vi "PH_Timing.calc GateGen Settings.vi"(5 "T2 [s]":i16 min=0 max=3000 step=100) -> (20 "Width Gate":dbl, 22 "Width T2":dbl, 24 "Delay Gate":dbl, 26 "Delay T2":dbl)   [LabVIEW 2014, in "PH_Timing.lvlib"]
doc: "This VI calculates the GateGen settings"
uses:
  PH_Timing.lvlib
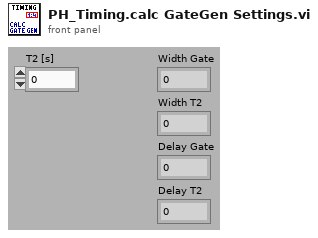
[diagram p1: front panel]
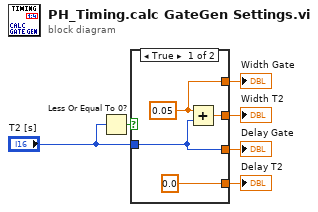
[diagram p0: block diagram]
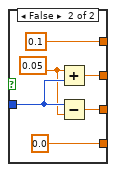
[diagram p2: hidden frame]
diagram:
  n1 = Less Or Equal To 0?(x="T2 [s]") -> (x <= 0?=w2:bool)
  n2 = case shown="True" w2 {
    tunnel: [w8 0.1 ("Gate Generator Settings.Width Single Shot")] -> w6
    tunnel: [w10 w14] -> w5
    tunnel: "T2 [s]" -> [w7 w13]
    tunnel: [0.0 ("Delay T2") 0.0 ("Delay T2")] -> w4
    tunnel: [w7 w11] -> w3
    frame True {
      w8 = 0.05 ("Gate Generator Settings.Width Single Shot")
      n3 = Add(x=w8, y=w7) -> (x+y=w10:dbl)
    }
    frame False {
      w12 = 0.05 ("Gate Generator Settings.Width Single Shot")
      n4 = Add(x=w12, y=w13) -> (x+y=w14:dbl)
      n5 = Subtract(x=w13, y=w12) -> (x-y=w11:dbl)
    }
  }
  "Width Gate" <- w6
  "Width T2" <- w5
  "Delay Gate" <- w3
  "Delay T2" <- w4
